vi "Read Commit Feed Folderpaths.vi"(8 "error in (no error)":errorcluster, 11 "CommitNIPKG_LV in":refnum<class "CommitNIPKG_LV.lvclass">) -> (0 "error out":errorcluster, 2 "Commit Feed Folderpaths":path[](array[path]), 3 "CommitNIPKG_LV out":refnum<class "CommitNIPKG_LV.lvclass">)   [LabVIEW 2017, in "CL_G3_VIComponentBuilder.lvlib" / "CommitNIPKG_LV.lvclass"]
uses:
  CommitNIPKG_LV.lvclass
  CommitNIPKG_LV.lvclass/CommitNIPKG_LV.ctl
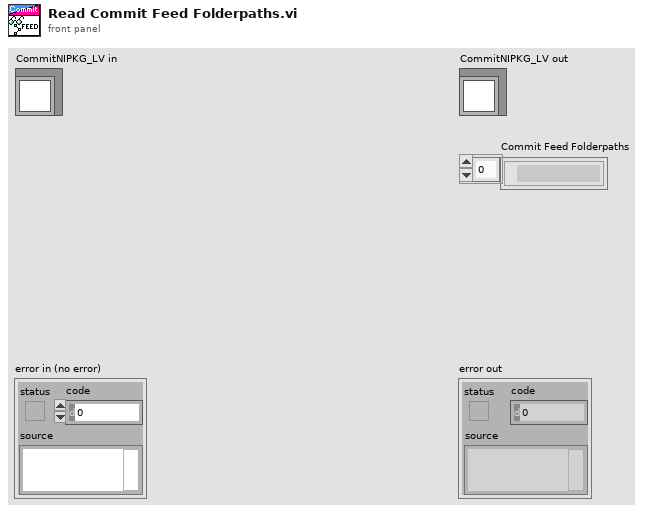
[diagram p1: front panel]
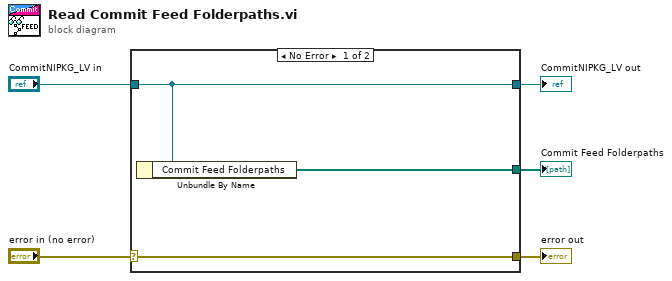
[diagram p0: block diagram]
diagram:
  n1 = case shown="No Error" "error in (no error)" {
    selector: "error in (no error)" -> [w8 w9]
    tunnel: [w8 w9] -> w4
    tunnel: [w7 w10] -> w2
    tunnel: "CommitNIPKG_LV in" -> [w7 w10]
    tunnel: [w6 _] -> w1
    frame No Error {
      n2 = Unbundle By Name(w7) -> ("Commit Feed Folderpaths"=w6:path[])
    }
    frame Error {
    }
  }
  "error out" <- w4
  "CommitNIPKG_LV out" <- w2
  "Commit Feed Folderpaths" <- w1
